vi "Top IO.vi"(7 "Object in":refnum<class>, 11 "String in":string) -> (3 "String out":string, 5 "Object out":refnum<class>)   [LabVIEW 2020]
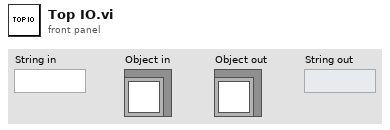
[diagram p1: front panel]
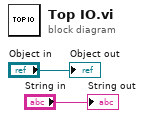
[diagram p0: block diagram]
diagram:
  "Object out" <- "Object in"
  "String out" <- "String in"
